vi "PH_Cont-601k_PowerUnit.PC PU on.vi"(0 "i ref in":refnum<vi>, 2 "PU on":bool, 5 "error in (no error)":errorcluster) -> (14 "i ref out":refnum<vi>, 19 "error out":errorcluster)   [LabVIEW 2014, in "PH_Cont-601k_PowerUnit.lvlib"]
doc: "This is the action VI of the PU on event case. Depending on the inout it does the following:\n\nfalse: set save state\ntrue: if the PreAmp is not disabled and State SM = \"Stand by\", a state change request is send to SM to get \"Switch PU on\" and the attribute \"PU in use\" is set to true. \nelse: GUI Knob is resetted"
uses:
  PH_Cont-601k_PowerUnit.lvlib
  PH_PowerUnit_BaseClass/PH_PowerUnit_BaseClass.lvlib
  PH_Cont-601k_PSU/PH_Cont-601k_PSU.lvlib
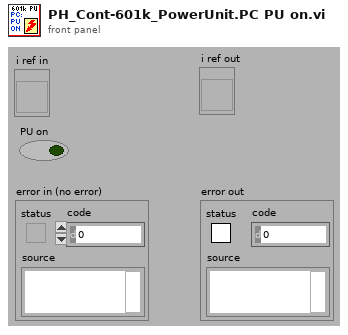
[diagram p1: front panel]
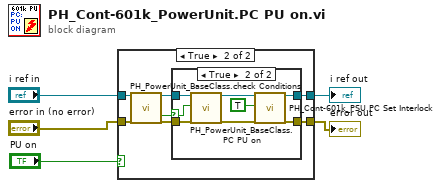
[diagram p0: block diagram]
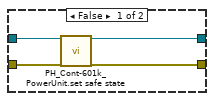
[diagram p2: hidden frame]
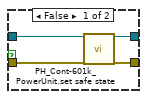
[diagram p3: hidden frame]
diagram:
  n1 = case shown="True" "PU on" {
    tunnel: "i ref in" -> [w9 w14]
    tunnel: [w8 w15] -> w5
    tunnel: "error in (no error)" -> [w7 w13]
    tunnel: [w6 w16] -> w4
    frame False {
      n2 = call "PH_Cont-601k_PowerUnit.set safe state.vi"("i ref in"=w9, "error in (no error)"=w7) -> ("i ref out"=w8:refnum<vi>, "error out"=w6:errorcluster)  [unwired: 16 in]
    }
    frame True {
      n3 = call "PH_PowerUnit_BaseClass.check Conditions.vi"("VI in"=w14, "error in (no error)"=w13) -> ("VI out"=w11:refnum<vi>, "Ready to switch PU on"=w12:bool, "error out"=w10:errorcluster)  [unwired: 14 in, 1 out]
      n4 = case shown="True" w12 {
        selector: w12 -> [_ w23]
        tunnel: [w17 w21] -> w16
        tunnel: [w19 w22] -> w15
        tunnel: w10 -> [w18 w26]
        tunnel: w11 -> [w20 w27]
        frame False {
          n5 = call "PH_Cont-601k_PowerUnit.set safe state.vi"("i ref in"=w20, "error in (no error)"=w18) -> ("i ref out"=w19:refnum<vi>, "error out"=w17:errorcluster)  [unwired: 16 in]
        }
        frame True {
          n6 = call "PH_PowerUnit_BaseClass.PC PU on.vi"("i ref in"=w27, "PU on"=w23, "error in (no error)"=w26) -> ("i ref out"=w25:refnum<vi>, "error out"=w24:errorcluster)  [unwired: 15 in]
          n7 = call "PH_Cont-601k_PSU.PC Set Interlock.vi"("VI in"=w25, "Set Interlock"=TRUE, "error in (no error)"=w24) -> ("VI out"=w22:refnum<vi>, "error out"=w21:errorcluster)  [unwired: 15 in]
        }
      }
    }
  }
  "error out" <- w4
  "i ref out" <- w5
